vi "CryoCoolerAVC Alarm Check.vi"(8 "error in (no error)":errorcluster, 9 "Cryo Alarms":T1, 10 "Cryocooler":string, 11 "CryoCooler Status":T3) -> (0 "error out":errorcluster, 1 "Alarms":T2[](array[typedef]), 2 "Message":string, 3 "alarm":bool, 4 "Shutdown?":bool)   [LabVIEW 2024]
uses:
  Cryo Cooler/CryoCoolerAVC/CryoCoolerAVC Status Cluster.ctl
  typedefs/CC cluster Alarm Data.ctl
  CryoCooler cluster Alarm Settings.ctl
  WebRelay10 Driver/CC WebRelay enum Actions.ctl
  Cryo Cooler/CryoCoolerAVC/CryoCoolerAVC.lvclass
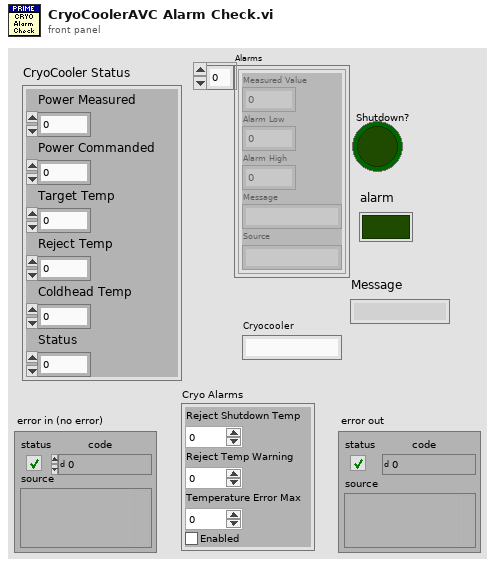
[diagram p1: front panel]
types:
  T1 = typedef "CryoCooler cluster Alarm Settings.ctl" = cluster{"Reject Shutdown Temp":dbl, "Reject Temp Warning":dbl, "Temperature Error Max":dbl, "Enabled":bool}
  T2 = typedef "CC cluster Alarm Data.ctl" = cluster{"Measured Value":dbl, "Alarm Low":dbl, "Alarm High":dbl, "Message":string, "Source":string}
  T3 = typedef "CryoCoolerAVC.lvclass/CryoCoolerAVC Status Cluster.ctl" = cluster{"Power Measured":dbl, "Power Commanded":dbl, "Target Temp":dbl, "Reject Temp":dbl, "Coldhead Temp":dbl, "Status":dbl}
  T4 = typedef "CC WebRelay enum Actions.ctl" = enum16{"Init", "Read Status", "Set Relay", "Close"}
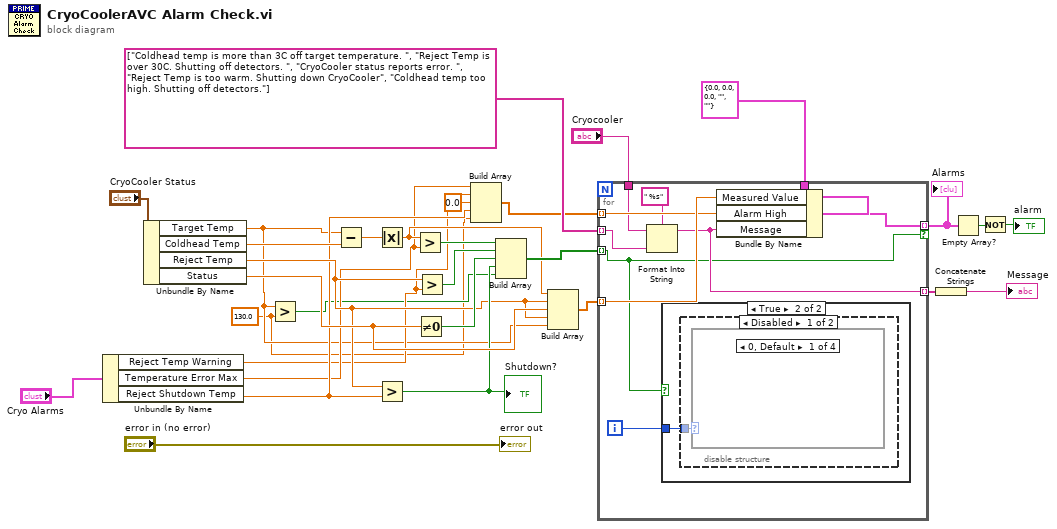
[diagram p0: block diagram]
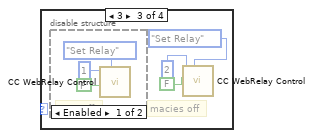
[diagram p4: hidden frame]
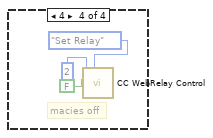
[diagram p6: hidden frame]
diagram:
  w1 = 130.0 ("y")
  n1 = Unbundle By Name("Cryo Alarms") -> ("Reject Temp Warning"=w4:dbl, "Temperature Error Max"=w5:dbl, "Reject Shutdown Temp"=w6:dbl)
  n2 = Unbundle By Name("CryoCooler Status") -> ("Target Temp"=w3:dbl, "Coldhead Temp"=w28:dbl, "Reject Temp"=w7:dbl, "Status"=w16:dbl)
  n3 = Greater?(x=w3, y=w1) -> (0:w2:bool)
  n4 = Subtract(x=w3, y=w28) -> (x-y=w27:dbl)
  n5 = Absolute Value(x=w27) -> (abs(x)=w17:dbl)
  n6 = Greater?(x=w7, y=w6) -> (0:w8:bool)
  "Shutdown?" <- w8
  n7 = Greater?(x=w17, y=w5) -> (0:w26:bool)
  n8 = Not Equal To 0?(x=w16) -> (x != 0?=w24:bool)
  n9 = Greater?(x=w7, y=w4) -> (0:w25:bool)
  n10 = Build Array(w5, w4, 0.0 ("element"), w6, w1) -> (w13:dbl[])
  n11 = Build Array(w26, w25, w24, w8, w2) -> (w23:bool[])
  n12 = Build Array(w17, w7, w16, w7, w3) -> (w15:dbl[])
  n13 = for {
    tunnel: w23 -> [w31] mode=indexing
    tunnel: string[] ["Coldhead temp is more than 3C off target temperature. ", "Reject Temp is over 30C. Shutting off detectors. ", "CryoCooler status reports error. ", "Reject Temp is too warm. Shutting down CryoCooler", "Coldhead temp too high. Shutting off detectors."] -> [w35] mode=indexing
    tunnel: [w39] -> w21 mode=indexing if=w31
    tunnel: T2 {"Measured Value"=0.0, "Alarm Low"=0.0, "Alarm High"=0.0, "Message"="", "Source"=""} -> [w40]
    tunnel: w15 -> [w38] mode=indexing
    tunnel: w13 -> [w37] mode=indexing
    tunnel: [w33] -> w12 mode=indexing
    tunnel: "Cryocooler" -> [w34]
    i -> [w32]
    n14 = Format Into String(format string=" %s", initial string=w34, w35) -> (resulting string=w33:string)  [unwired: 1 in, 1 out]
    n15 = case shown="True" w31 {
      tunnel: w32 -> [_ w41]
      frame False {
      }
      frame True {
        n16 = disable-structure shown="Disabled" {
          disable-tunnel: w41 -> [w42 _]
          frame Disabled {
            n17 = case shown="0, Default" w42 {
              frame 0, Default {
              }
              frame 1 {
              }
              frame 3 {
                # "macies off"
                n18 = disable-structure shown="Enabled" {
                  frame Enabled {
                    # "Cryo off"
                    n19 = call "CC WebRelay Control.vi"("Action"=CC_WebRelay_enum_Actions."Set Relay", "state"=FALSE, "Relay (1 to 10)"=1) -> ()  [unwired: 7 in, 2 out]
                  }
                  frame Disabled {
                  }
                }
                n20 = call "CC WebRelay Control.vi"("Action"=CC_WebRelay_enum_Actions."Set Relay", "state"=FALSE, "Relay (1 to 10)"=2) -> ()  [unwired: 7 in, 2 out]
              }
              frame 4 {
                # "macies off"
                n21 = call "CC WebRelay Control.vi"("Action"=CC_WebRelay_enum_Actions."Set Relay", "state"=FALSE, "Relay (1 to 10)"=2) -> ()  [unwired: 7 in, 2 out]
              }
            }
          }
          frame Enabled {
          }
        }
      }
    }
    n22 = Bundle By Name(cluster=w40, "Measured Value"=w38, "Alarm High"=w37, "Message"=w33) -> (w39:T2)
  }
  "Alarms" <- w21
  n23 = Concatenate Strings(w12) -> (→"Message":string)
  n24 = Empty Array?(array=w21) -> (empty?=w19:bool)
  n25 = Not(x=w19) -> (.not. x?=→"alarm":bool)
  "error out" <- "error in (no error)"
